vi "SR_FlipFlopWithClear.vi"(0 "_____\nClear":bool, 3 "R":bool, 4 "CLK":bool, 5 "S":bool, 6 "________\nPresent":bool) -> (1 "__\nQ":bool, 2 "Q":bool)   [LabVIEW 2018]
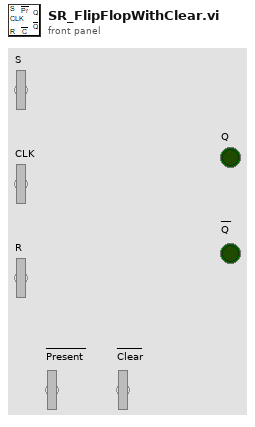
[diagram p1: front panel]
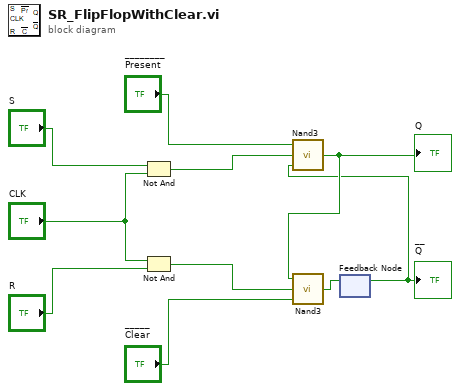
[diagram p0: block diagram]
diagram:
  n1 = Not And(1:"CLK", 2:"S") -> (0:w7:bool)
  n2 = Not And(1:"R", 2:"CLK") -> (0:w6:bool)
  n3 = feedback #1() -> (w1:bool)  [unwired: 1 in]
  "__\nQ" <- w1
  n4 = call "Nand3.vi"("C"=w1, "B"=w7, "A"="________\nPresent") -> ("Boolean"=w3:bool)
  "Q" <- w3
  n5 = call "Nand3.vi"("C"="_____\nClear", "B"=w6, "A"=w3) -> ("Boolean"=w2:bool)
  n6 = feedback-in #1(w2) -> ()
